vi "Stoerungen (129-192)- Messgeraet.vi"(8 "Fehler (Eingang)":errorcluster caption="Fehler (Eingang, kein Fehler)") -> (0 "Fehler (Ausgang)":errorcluster, 3 "Störungen 129-192":u64)   [LabVIEW 2020, in "Stoerungen.lvlib"]
uses:
  Stoerungen.lvlib
  Seiten/FT-IR/FGV FT-IR Diagnose Aktionen.ctl
  cRIO/Stoermeldungen/Stoerungen 129-192.ctl
  Aktionen Kommunikation Stoerung.ctl
  Seiten/Anlagengrenzwerte/Anlagen-Parameternamen.ctl
  Seiten/Erweiterte Konfig/FGV PID Aktionen.ctl
  Seiten/FT-IR/FGV FT-IR Aktionen.ctl
  Seiten/Log Konfig/Aktionen LogFile schreiben.ctl
  Funktionstasten/Funktionstasten-Aktion.ctl
  Funktionstasten/Zustaende.ctl
  Status Analysatoren/Aktion Status Analysatoren.ctl
  Seiten/EL3000/PMA/Aktion FGV Messwerte.ctl
  Seiten/EL3000/FID/Aktion FGV Messwerte_F.ctl
  Allgemein/Aktion FGV Aufheizphase.ctl
  Seiten/Lambdasonde/FGV Status Lambda Aktionen.ctl
  Seiten/FT-IR/FT-IR.lvlib
  cRIO/Stoermeldungen/Stoermeldungen.lvlib
  Seiten/Anlagengrenzwerte/Anlagengrenzwerte.lvlib
  Seiten/Erweiterte Konfig/Erweiterte Konfig.lvlib
  Seiten/Log Konfig/LogKonfig.lvlib
  cRIO/PC/Kommunikation mit cRIO.lvlib
  Funktionstasten/Funktionstasten.lvlib
  Status Analysatoren/Status Analysatoren.lvlib
  Seiten/EL3000/PMA/PMA.lvlib
  Seiten/EL3000/FID/FID.lvlib
  Seiten/Lambdasonde/Lambda_ Komm.lvlib
  Allgemein/allgemeine Sub-VIs.lvlib
panel:
  # "Störmeldungen Messgerät (129-192)"
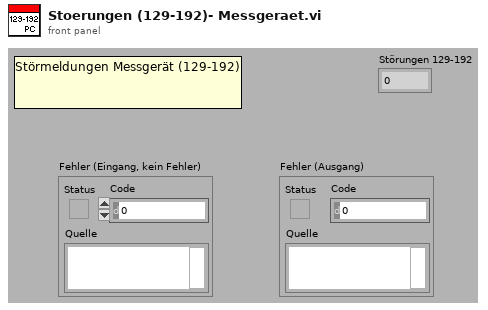
[diagram p1: front panel]
types:
  T1 = typedef "allgemeine Sub-VIs.lvlib/Aktion FGV Aufheizphase.ctl" = enum16{"init", "lesen", "PNS Filterblock", "PNS HL1", "PNS HL2", "PNS HL3", "PNS HL4", "FTIR Messzelle", "HL 1", "HL 2", "HL zu FTIR", "auswerten"}
  T2 = typedef "Status Analysatoren.lvlib/Aktion Status Analysatoren.ctl" = enum16{"lesen", "initialisieren", "Analysatoren aktiv", "FTIR Fehler", "FID Fehler", "PMA Fehler", "Felder einfärben"}
  T3 = typedef "ABB-EL3000.lvlib/FID.lvlib/Aktion FGV Messwerte_F.ctl" = enum16{"lesen", "Messwerte", "Messbereich", "Status", "Diagnose Werte"}
  T4 = typedef "ABB-EL3000.lvlib/PMA.lvlib/Aktion FGV Messwerte.ctl" = enum16{"lesen", "Messwerte", "Messbereich", "Status", "Diagnose Werte"}
  T5 = typedef "Funktionstasten.lvlib/Zustaende.ctl" = enum16{"Standby", "Pause", "Eco", "Messen", "Kalibrieren", "Spülen Filter", "Spülen Leitung", "Umgebungsluft", "0-Gas", "Cal-Gas", "CG zu PNS", "-------------", "Init 1", "Init 2", "Init 3", "Init 4", "Messen vorbereiten", "Messen durchführen", "Exit"}
  T6 = typedef "Funktionstasten.lvlib/Funktionstasten-Aktion.ctl" = enum16{"Initialisieren", "Zustand setzen", "Taste gedrückt", "Fehler speichern", "Lesen", "Manuell", "Remote", "Bitparallel", "Samplepoint", "Zeit Prüfen", "reset Umschalten"}
  T7 = typedef "LogKonfig.lvlib/Aktionen LogFile schreiben.ctl" = enum16{"lesen", "schreiben", "initialisieren"}
  T8 = typedef "FT-IR.lvlib/FGV FT-IR Aktionen.ctl" = enum16{"lesen", "NOG setzen", "NOS setzen", "Initialisieren", "speichern", "ALLES setzen", "FT-IR Spektrum loggen", "Komm Stoppen", "Spektrum LogKonfig"}
  T9 = typedef "Erweiterte Konfig.lvlib/FGV PID Aktionen.ctl" = enum16{"Lesen", "Schreiben PID", "Schreiben Sonstige", "Dichtheitstest", "Aktionen Dicht.", "Parameter Sensor"}
  T10 = typedef "Stoerungen.lvlib/Aktionen Kommunikation Stoerung.ctl" = enum16{"lesen", "init", "FT-IR Komm", "FT-IR Betriebsart", "FT-IR Hintergrund", "cRIO Komm", "PNS Komm", "Dichtheitstest", "Life Bit", "FTIR Komm AK", "PMA Komm", "FID Komm", "PMA Cal", "FID Ch4 Cal", "FID THC Cal", "Cal Timeout", "VFS 1 Komm", "VFS 2 Komm", "VFS 3 Komm", "VFS 4 Komm", "TRE 08 Komm", "CG-Test vorzeitig", "CG-Test Span 1", "CG-Test Span 2", "CG-Test Span 3", "CG-Test Messgas", "CG-Test löschen", "Test", "Amium AK", "AK Recept konfig", "AK Name konfig", "AK EKFG konfig"}
  T11 = typedef "Anlagengrenzwerte.lvlib/Anlagen-Parameternamen.ctl" = enum16{"Eingangsdruck FT-IR:", "Durchfluss FT-IR:", "Durchfluss CalGas", "Druck Ausgang", "Druck Kalter Block", "Heizleitung intern", "Heizleitung zu FT-IR", "Heizung Filter:", "Heizung Pumpe:", "HL Extern SP1", "HL Extern SP2", "FT-IR Messzelle", "Schaltschrank", "Gaskühler"}
  T12 = typedef "Stoermeldungen.lvlib/Stoerungen 129-192.ctl" = cluster{"ERR. 129":bool, "ERR. 130":bool, "ERR. 131":bool, "ERR. 132":bool, "ERR. 133":bool, "ERR. 134":bool, "ERR. 135":bool, "ERR. 136":bool, "ERR. 137":bool, "ERR. 138":bool, "ERR. 139":bool, "ERR. 140":bool, "ERR. 141":bool, "ERR. 142":bool, "ERR. 143":bool, "ERR. 144":bool, "ERR. 145":bool, "ERR. 146":bool, "ERR. 147":bool, "ERR. 148":bool, "ERR. 149":bool, "ERR. 150":bool, "ERR. 151":bool, "ERR. 152":bool, "ERR. 153":bool, "ERR. 154":bool, "ERR. 155":bool, "ERR. 156":bool, "ERR. 157":bool, "ERR. 158":bool, "ERR. 159":bool, "ERR. 160":bool, "ERR. 161":bool, "ERR. 162":bool, "ERR. 163":bool, "ERR. 164":bool, "ERR. 165":bool, "ERR. 166":bool, "ERR. 167":bool, "ERR. 168":bool, "ERR. 169":bool, "ERR. 170":bool, "ERR. 171":bool, "ERR. 172":bool, "ERR. 173":bool, "ERR. 174":bool, "ERR. 175":bool, "ERR. 176":bool, "ERR. 177":bool, "ERR. 178":bool, "ERR. 179":bool, "ERR. 180":bool, "ERR. 181":bool, "ERR. 182":bool, "ERR. 183":bool, "ERR. 184":bool, "ERR. 185":bool, "ERR. 186":bool, "ERR. 187":bool, "ERR. 188":bool, "ERR. 189":bool, "ERR. 190":bool, "ERR. 191":bool, "ERR. 192":bool}
  T13 = typedef "FT-IR.lvlib/FGV FT-IR Diagnose Aktionen.ctl" = enum16{"Lesen", "Diagnose Schreiben", "Min Schreiben", "Max Schreiben"}
  T14 = typedef "Stoerungen.lvlib/Stoerungen Messgeraete.ctl" = cluster{"FT-IR Komm":bool, "FT-IR Betriebsart":bool, "FT-IR Hintergrundscan":bool, "Dichtheitstest":bool, "cRIO Komm":bool, "PNS Komm":bool, "Life Bit":bool, "FT-IR AK Komm":bool, "PMA Komm":bool, "FID Komm":bool, "PMA Cal":bool, "FID CH4 Cal":bool, "FID THC Cal":bool, "Cal Timeout":bool, "VFS 1 Komm":bool, "VFS 2 Komm":bool, "VFS 3 Komm":bool, "VFS 4 Komm":bool, "TRE 08 Komm":bool, "CG-Test":bool, "CG-Test 1":bool, "CG-Test 2":bool, "CG-Test 3":bool, "Messgas - Eingang":bool, "Amium AK Komm":bool, "AK Rezept nicht konfiguriert ":bool, "AK Name nicht konfiguriert":bool, "AK EKFG nicht konfiguriert":bool}
  T15 = cluster{"LaserPP Max":dbl, "LinCheck Max":dbl, "sBeam Max":dbl}
  T16 = cluster{"LaserPP Min":dbl, "LinCheck Min":dbl, "sBeam Min":dbl}
  T17 = typedef "FT-IR.lvlib/TOOLweb Interface.lvlib/Typdefinitionen.lvlib/TOOLweb Diagnose.ctl" = cluster{"(14) temperature":sgl, "(15) pressure":sgl, "(16) oxygen":sgl, "(50) diag-igramdc":sgl, "(51) diag-igrampp":sgl, "(52) diag-phaseAngle":sgl, "(53) diag-laserpp":sgl, "(54) diag-laserdc":sgl, "(55) diag-badscan":sgl, "(56) diag-centerburst":sgl, "(57) diag-linearizerCheck":sgl, "(58) diag-SNR":sgl, "(59) diag-sBeamIntensity":sgl}
  T18 = typedef "Verwaltung - cRIO.lvlib/Digital Eingaenge 0-15.ctl" = cluster{"I0: N2 Nachf. FT-IR voll":bool, "I1: N2 Nachf. Vorrat leer":bool, "I2: (Klimaanlage eingeschaltet)":bool, "I3: (Klimaanlage Störung)":bool, "I4: Trigger Eingang (Messdaten sp.)":bool, "I5: Reserve":bool, "I6: Reserve":bool, "I7: Reserve":bool, "I8: Druckschalter Versorgung ok":bool, "I9: Reserve":bool, "I10: Reserve":bool, "I11: Reserve":bool, "I12: Drucksch. N2 Versorgung":bool, "I13: Reserve":bool, "I14: Drucksch. N2 Optikbox":bool, "I15: (Füllstand Kondensatbehälter)":bool}
  T19 = typedef "Status Analysatoren.lvlib/Status.ctl" = cluster{"FT-IR aktiv":bool, "FT-IR Fehler":bool, "FID aktiv":bool, "FID Fehler":bool, "PMA aktiv":bool, "PMA Fehler":bool}
  T20 = cluster{"Temperatur Detektor":sgl, "STG Detektor":sgl, "Temperatur MGE":sgl, "STG MGE":sgl, "Druck Brennluft":sgl, "STG Brennluft":sgl, "Druck Brenngas":sgl, "STG Brenngas":sgl, "Druck MGE":sgl, "STG Druck MGE":sgl, "Druck MGA":sgl, "STG Druck MGA":sgl, "Flow":sgl, "Temperatur Flamme":sgl, "Temperatur NMHC":sgl, "STG NMHC":sgl}
  T21 = cluster{"Ausfall":bool, "Funktionskontrolle":bool, "Wartungsbedarf":bool}
  T22 = cluster{"Temp. Detektor":sgl, "Temp. Regler":sgl, "STG Regler":sgl, "Druck Detektor":sgl}
  T23 = typedef "Erweiterte Konfig.lvlib/Sonstige Parameter.ctl" = cluster{"Lüfter langsam":sgl, "Lüfter schnell":sgl, "FT-IR Kühlung Soll":sgl, "FT-IR Kühlung Max":sgl, "Überwachung":T24, "Befüllung aktiv":T25, "Stickstoff Befüllzeit":sgl, "Befüllintervall":sgl, "Kalibrierwert FT-IR":sgl, "Offset Ausgang":sgl, "Offset FT-IR":sgl, "Offset Druck FT-IR":sgl, "Dichtheitstest Zeit":sgl, "Dichtheitstest Abfall":sgl, "Dichtheitstest Umfang":T26, "Offset Umgebung":sgl, "Max Taupunkt":sgl, "Pumpendrehzahl":sgl, "ext. Befüllung":T25, "Ext. Stickstoff Befüllzeit":sgl}
  T24 = typedef "Auswahlfeld.ctl" = u16
  T25 = typedef "LogKonfig.lvlib/Auswahlfeld aktiviert-deaktiviert.ctl" = u16
  T26 = typedef "Erweiterte Konfig.lvlib/Dichtheitstest Umfang.ctl" = u16
  T27 = typedef "Lambda_ Komm.lvlib/FGV Status Lambda Aktionen.ctl" = enum16{"lesen", "init", "Istwerte"}
  T28 = typedef "Lambda_ Komm.lvlib/Lambda Fehler.ctl" = cluster{"Komm":bool, "Lambda  Fehler":bool, "Ri Fehler":bool, "O2 Fehler":bool, "A/F Fehler":bool}
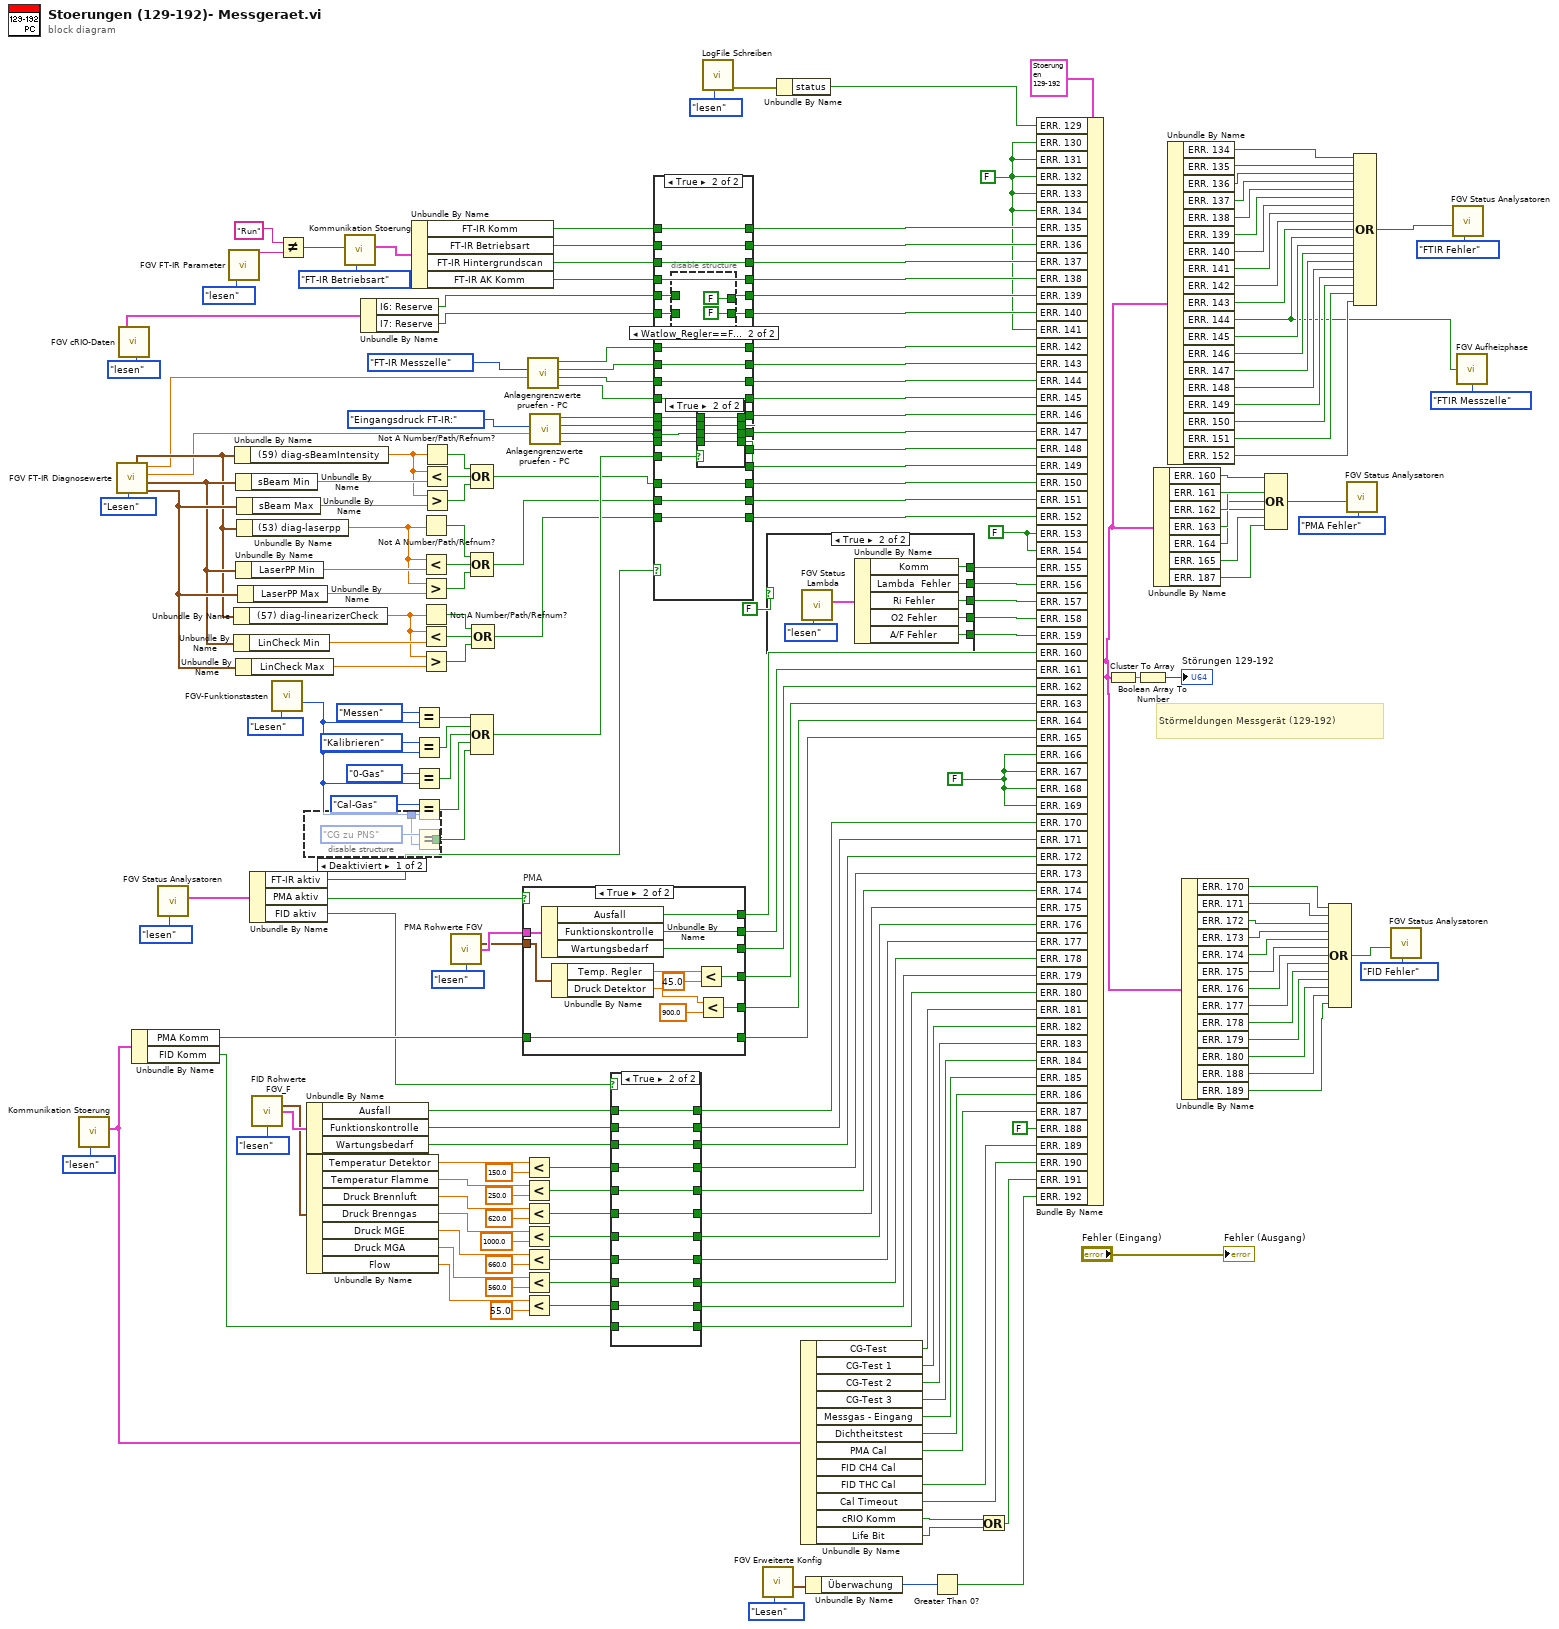
[diagram p0: block diagram]
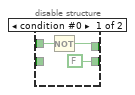
[diagram p7: hidden frame]
diagram:
  w16 = FALSE ("ERR. 173")
  w119 = FALSE ("ERR. 129")
  w67 = FALSE ("ERR. 129")
  # "Störmeldungen Messgerät (129-192)"
  n1 = call "Kommunikation Stoerung.vi"("Aktionen"=Aktionen_Kommunikation_Stoerung."lesen") -> ("Störung Messgerät"=w109:T14)  [unwired: 10 in]
  n2 = call "FGV FT-IR Diagnosewerte.vi"("Aktionen"=FGV_FT-IR_Diagnose_Aktionen."Lesen") -> ("FT-IR MAX"=w212:T15, "FT-IR MIN"=w211:T16, "Druck"=w202:dbl, "Temperatur"=w203:dbl, "Diagnose"=w210:T17)  [unwired: 5 in, 1 out]
  n3 = call "FGV cRIO-Daten.vi"("Aktion"=enum16{"lesen", "schreiben"}."lesen") -> ("DI"=w171:T18)  [unwired: 9 in, 9 out]
  n4 = Unbundle By Name(w109) -> ("PMA Komm"=w108:bool, "FID Komm"=w79:bool)
  n5 = call "FGV Status Analysatoren.vi"("Aktionen"=Aktion_Status_Analysatoren."lesen") -> ("Status Analysatoren"=w121:T19)  [unwired: 10 in]
  n6 = call "FGV FT-IR Parameter.vi"("Aktion"=FGV_FT-IR_Aktionen."lesen") -> ("Instrument State"=w189:string)  [unwired: 11 in, 7 out]
  n7 = Unbundle By Name(w210) -> ("(57) diag-linearizerCheck"=w178:sgl)
  n8 = Unbundle By Name(w211) -> ("LinCheck Min"=w206:dbl)
  n9 = Unbundle By Name(w210) -> ("(59) diag-sBeamIntensity"=w184:sgl)
  n10 = Unbundle By Name(w211) -> ("sBeam Min"=w214:dbl)
  n11 = Unbundle By Name(w211) -> ("LaserPP Min"=w209:dbl)
  n12 = Unbundle By Name(w212) -> ("LinCheck Max"=w207:dbl)
  n13 = Unbundle By Name(w212) -> ("sBeam Max"=w215:dbl)
  n14 = Unbundle By Name(w210) -> ("(53) diag-laserpp"=w179:sgl)
  n15 = Unbundle By Name(w212) -> ("LaserPP Max"=w208:dbl)
  n16 = Unbundle By Name(w121) -> ("FT-IR aktiv"=w120:bool, "PMA aktiv"=w21:bool, "FID aktiv"=w80:bool)
  n17 = call "FID Rohwerte FGV_F.vi"("Aktion"=Aktion_FGV_Messwerte_F."lesen") -> ("Diagnose Werte"=w102:T20, "Status"=w106:T21)  [unwired: 11 in, 2 out]
  n18 = call "FGV-Funktionstasten.vi"("Aktion"=Funktionstasten-Aktion."Lesen") -> ("ausgewählte Funktion"=w3:T5)  [unwired: 7 in, 7 out]
  n19 = Not Equal?(x="Run" ("y"), y=w189) -> (x != y?=w188:bool)
  n20 = disable-structure shown="Deaktiviert" {
    disable-tunnel: w3 -> [w218 _]
    disable-tunnel: [w217 _] -> w156
    frame Disabled {
      n21 = Equal?(x=Zustaende."CG zu PNS", y=w218) -> (x = y?=w217:bool)
    }
    frame Enabled {
    }
  }
  n22 = Unbundle By Name(w106) -> ("Ausfall"=w105:bool, "Funktionskontrolle"=w104:bool, "Wartungsbedarf"=w103:bool)
  n23 = Unbundle By Name(w102) -> ("Temperatur Detektor"=w101:sgl, "Temperatur Flamme"=w100:sgl, "Druck Brennluft"=w99:sgl, "Druck Brenngas"=w98:sgl, "Druck MGE"=w97:sgl, "Druck MGA"=w96:sgl, "Flow"=w95:sgl)
  n24 = call "Kommunikation Stoerung.vi"("Aktionen"=Aktionen_Kommunikation_Stoerung."FT-IR Betriebsart", "ERROR"=w188) -> ("Störung Messgerät"=w199:T14)  [unwired: 9 in]
  n25 = Unbundle By Name(w171) -> ("I6: Reserve"=w170:bool, "I7: Reserve"=w169:bool)
  n26 = Unbundle By Name(w199) -> ("FT-IR Komm"=w155:bool, "FT-IR Betriebsart"=w153:bool, "FT-IR Hintergrundscan"=w151:bool, "FT-IR AK Komm"=w149:bool)
  n27 = Equal?(x=Zustaende."Messen", y=w3) -> (x = y?=w160:bool)
  n28 = Equal?(x=Zustaende."Kalibrieren", y=w3) -> (x = y?=w159:bool)
  n29 = Equal?(x=Zustaende."0-Gas", y=w3) -> (x = y?=w158:bool)
  n30 = Equal?(x=Zustaende."Cal-Gas", y=w3) -> (x = y?=w157:bool)
  n31 = Not A Number/Path/Refnum?(number/path/refnum=w179) -> (NaN/Path/Refnum?=w183:bool)
  n32 = Less?(x=w179, y=w209) -> (x < y?=w182:bool)
  n33 = Greater?(x=w179, y=w208) -> (0:w176:bool)
  n34 = Not A Number/Path/Refnum?(number/path/refnum=w178) -> (NaN/Path/Refnum?=w181:bool)
  n35 = Less?(x=w178, y=w206) -> (x < y?=w180:bool)
  n36 = Greater?(x=w178, y=w207) -> (0:w177:bool)
  n37 = Not A Number/Path/Refnum?(number/path/refnum=w184) -> (NaN/Path/Refnum?=w185:bool)
  n38 = Less?(x=w184, y=w214) -> (x < y?=w187:bool)
  n39 = Greater?(x=w184, y=w215) -> (0:w186:bool)
  n40 = call "PMA Rohwerte FGV.vi"("Aktion"=Aktion_FGV_Messwerte."lesen") -> ("Diagnose Werte"=w116:T22, "Status"=w117:T21)  [unwired: 11 in, 2 out]
  n41 = Compound Arithmetic op=OR(w185, w187, w186) -> (w127:bool)
  n42 = Compound Arithmetic op=OR(w183, w182, w176) -> (w125:bool)
  n43 = Compound Arithmetic op=OR(w160, w159, w158, w157, w156) -> (w133:bool)
  n44 = Compound Arithmetic op=OR(w181, w180, w177) -> (w123:bool)
  n45 = case "PMA" shown="True" w21 {
    tunnel: w117 -> [_ w231]
    tunnel: w116 -> [_ w230]
    tunnel: [_ w225] -> w112
    tunnel: [_ w224] -> w111
    tunnel: [_ w223] -> w115
    tunnel: [_ w222] -> w114
    tunnel: [_ w221] -> w113
    tunnel: w108 -> [_ w220]
    tunnel: [_ w220] -> w110
    frame False {
    }
    frame True {
      n46 = Unbundle By Name(w231) -> ("Ausfall"=w223:bool, "Funktionskontrolle"=w222:bool, "Wartungsbedarf"=w221:bool)
      n47 = Unbundle By Name(w230) -> ("Temp. Regler"=w229:sgl, "Druck Detektor"=w226:sgl)
      n48 = Less?(x=w229, y=sgl 45.0) -> (x < y?=w225:bool)
      n49 = Less?(x=w226, y=sgl 900.0) -> (x < y?=w224:bool)
    }
  }
  n50 = Less?(x=w101, y=sgl 150.0) -> (x < y?=w87:bool)
  n51 = Less?(x=w100, y=sgl 250.0) -> (x < y?=w86:bool)
  n52 = Less?(x=w99, y=sgl 620.0) -> (x < y?=w85:bool)
  n53 = Less?(x=w98, y=sgl 1000.0) -> (x < y?=w84:bool)
  n54 = Less?(x=w97, y=sgl 660.0) -> (x < y?=w83:bool)
  n55 = Less?(x=w96, y=sgl 560.0) -> (x < y?=w82:bool)
  n56 = Less?(x=w95, y=sgl 55.0) -> (x < y?=w81:bool)
  n57 = call "Anlagengrenzwerte pruefen - PC.vi"("Wert"=w203, "Anlagen-Parametername"=Anlagen-Parameternamen."FT-IR Messzelle") -> ("AbschMax"=w138:bool, "AbschMin"=w140:bool, "WarnMax"=w142:bool, "WarnMin"=w144:bool)  [unwired: 5 in, 1 out]
  n58 = call "Anlagengrenzwerte pruefen - PC.vi"("Wert"=w202, "Anlagen-Parametername"=Anlagen-Parameternamen."Eingangsdruck FT-IR:") -> ("AbschMax"=w134:bool, "AbschMin"=w135:bool, "WarnMax"=w137:bool, "WarnMin"=w136:bool)  [unwired: 5 in, 1 out]
  n59 = case shown="True" w80 {
    tunnel: w105 -> [_ w237]
    tunnel: w104 -> [_ w236]
    tunnel: w103 -> [_ w235]
    tunnel: w87 -> [_ w234]
    tunnel: w86 -> [_ w233]
    tunnel: w85 -> [_ w232]
    tunnel: w84 -> [_ w238]
    tunnel: w83 -> [_ w239]
    tunnel: w82 -> [_ w240]
    tunnel: w81 -> [_ w241]
    tunnel: w79 -> [_ w242]
    tunnel: [_ w242] -> w68
    tunnel: [_ w241] -> w69
    tunnel: [_ w240] -> w70
    tunnel: [_ w239] -> w71
    tunnel: [_ w238] -> w72
    tunnel: [_ w237] -> w78
    tunnel: [_ w236] -> w77
    tunnel: [_ w235] -> w76
    tunnel: [_ w234] -> w75
    tunnel: [_ w233] -> w74
    tunnel: [_ w232] -> w73
    frame False {
    }
    frame True {
    }
  }
  n60 = case shown="True" w120 {
    tunnel: w155 -> [_ w266]
    tunnel: [_ w266] -> w154
    tunnel: w153 -> [_ w265]
    tunnel: [_ w265] -> w152
    tunnel: w151 -> [_ w264]
    tunnel: [_ w264] -> w150
    tunnel: w149 -> [_ w263]
    tunnel: [_ w263] -> w148
    tunnel: w170 -> [_ w244]
    tunnel: [_ w246] -> w147
    tunnel: w169 -> [_ w243]
    tunnel: [_ w245] -> w146
    tunnel: [_ w262] -> w145
    tunnel: w144 -> [_ w262]
    tunnel: w142 -> [_ w261]
    tunnel: [_ w261] -> w143
    tunnel: [_ w260] -> w141
    tunnel: w140 -> [_ w260]
    tunnel: [_ w259] -> w139
    tunnel: w138 -> [_ w259]
    tunnel: w136 -> [_ w258]
    tunnel: w137 -> [_ w257]
    tunnel: w135 -> [_ w256]
    tunnel: w134 -> [_ w255]
    tunnel: w133 -> [_ w254]
    tunnel: [_ w253] -> w132
    tunnel: [_ w252] -> w131
    tunnel: [_ w251] -> w130
    tunnel: [_ w250] -> w129
    tunnel: [_ w249] -> w128
    tunnel: w127 -> [_ w249]
    tunnel: [_ w248] -> w126
    tunnel: w125 -> [_ w248]
    tunnel: [_ w247] -> w124
    tunnel: w123 -> [_ w247]
    frame False {
    }
    frame True {
      n61 = disable-structure shown="Watlow_Regler==FALSE, Standard" {
        disable-tunnel: [w268 FALSE] -> w246
        disable-tunnel: [FALSE FALSE] -> w245
        disable-tunnel: w244 -> [w269 _]
        disable-tunnel: w243 -> [_ _]
        frame condition #0 {
          n62 = Not(x=w269) -> (.not. x?=w268:bool)
        }
        frame condition #1 (active) {
        }
      }
      n63 = case shown="True" w254 {
        tunnel: w258 -> [_ w272]
        tunnel: w257 -> [_ w273]
        tunnel: w256 -> [_ w274]
        tunnel: w255 -> [_ w275]
        tunnel: [_ w275] -> w250
        tunnel: [_ w274] -> w251
        tunnel: [_ w273] -> w252
        tunnel: [_ w272] -> w253
        frame False {
        }
        frame True {
        }
      }
    }
  }
  n64 = call "LogFile Schreiben.vi"("Aktion"=Aktionen_LogFile_schreiben."lesen") -> ("error out"=w173:errorcluster)  [unwired: 7 in, 3 out]
  n65 = call "FGV Erweiterte Konfig.vi"("Aktion"=FGV_PID_Aktionen."Lesen") -> ("Sonstige"=w195:T23)  [unwired: 6 in, 4 out]
  n66 = case shown="True" FALSE {
    tunnel: [_ w280] -> w66
    tunnel: [_ w279] -> w65
    tunnel: [_ w278] -> w64
    tunnel: [_ w277] -> w63
    tunnel: [_ w276] -> w62
    frame False {
    }
    frame True {
      n67 = call "FGV Status Lambda.vi"("Aktionen"=FGV_Status_Lambda_Aktionen."lesen") -> ("Lambda Fehler"=w282:T28)  [unwired: 9 in, 1 out]
      n68 = Unbundle By Name(w282) -> ("Komm"=w280:bool, "Lambda  Fehler"=w279:bool, "Ri Fehler"=w278:bool, "O2 Fehler"=w277:bool, "A/F Fehler"=w276:bool)
    }
  }
  n69 = Unbundle By Name(w173) -> ("status"=w175:bool)
  n70 = Unbundle By Name(w109) -> ("CG-Test"=w11:bool, "CG-Test 1"=w12:bool, "CG-Test 2"=w13:bool, "CG-Test 3"=w14:bool, "Messgas - Eingang"=w15:bool, "Dichtheitstest"=w17:bool, "PMA Cal"=w10:bool, "FID THC Cal"=w18:bool, "Cal Timeout"=w19:bool, "cRIO Komm"=w168:bool, "Life Bit"=w167:bool)  [unwired: 1 out]
  n71 = Unbundle By Name(w195) -> ("Überwachung"=w193:T24)
  n72 = Greater Than 0?(x=w193) -> (x > 0?=w192:bool)
  n73 = Or(x=w168, y=w167) -> (x .or. y?=w166:bool)
  n74 = Bundle By Name(cluster=T12 {"ERR. 129"=FALSE, "ERR. 130"=FALSE, "ERR. 131"=FALSE, "ERR. 132"=FALSE, "ERR. 133"=FALSE, "ERR. 134"=FALSE, "ERR. 135"=FALSE, "ERR. 136"=FALSE, "ERR. 137"=FALSE, "ERR. 138"=FALSE, "ERR. 139"=FALSE, "ERR. 140"=FALSE, "ERR. 141"=FALSE, "ERR. 142"=FALSE, "ERR. 143"=FALSE, "ERR. 144"=FALSE, "ERR. 145"=FALSE, "ERR. 146"=FALSE, "ERR. 147"=FALSE, "ERR. 148"=FALSE, "ERR. 149"=FALSE, "ERR. 150"=FALSE, "ERR. 151"=FALSE, "ERR. 152"=FALSE, "ERR. 153"=FALSE, "ERR. 154"=FALSE, "ERR. 155"=FALSE, "ERR. 156"=FALSE, "ERR. 157"=FALSE, "ERR. 158"=FALSE, "ERR. 159"=FALSE, "ERR. 160"=FALSE, "ERR. 161"=FALSE, "ERR. 162"=FALSE, "ERR. 163"=FALSE, "ERR. 164"=FALSE, "ERR. 165"=FALSE, "ERR. 166"=FALSE, "ERR. 167"=FALSE, "ERR. 168"=FALSE, "ERR. 169"=FALSE, "ERR. 170"=FALSE, "ERR. 171"=FALSE, "ERR. 172"=FALSE, "ERR. 173"=FALSE, "ERR. 174"=FALSE, "ERR. 175"=FALSE, "ERR. 176"=FALSE, "ERR. 177"=FALSE, "ERR. 178"=FALSE, "ERR. 179"=FALSE, "ERR. 180"=FALSE, "ERR. 181"=FALSE, "ERR. 182"=FALSE, "ERR. 183"=FALSE, "ERR. 184"=FALSE, "ERR. 185"=FALSE, "ERR. 186"=FALSE, "ERR. 187"=FALSE, "ERR. 188"=FALSE, "ERR. 189"=FALSE, "ERR. 190"=FALSE, "ERR. 191"=FALSE, "ERR. 192"=FALSE} ("STÖRUNGEN 129-192"), "ERR. 129"=w175, "ERR. 130"=w67, "ERR. 131"=w67, "ERR. 132"=w67, "ERR. 133"=w67, "ERR. 134"=w67, "ERR. 135"=w154, "ERR. 136"=w152, "ERR. 137"=w150, "ERR. 138"=w148, "ERR. 139"=w147, "ERR. 140"=w146, "ERR. 141"=w67, "ERR. 142"=w145, "ERR. 143"=w143, "ERR. 144"=w141, "ERR. 145"=w139, "ERR. 146"=w132, "ERR. 147"=w131, "ERR. 148"=w130, "ERR. 149"=w129, "ERR. 150"=w128, "ERR. 151"=w126, "ERR. 152"=w124, "ERR. 153"=w119, "ERR. 154"=w119, "ERR. 155"=w66, "ERR. 156"=w65, "ERR. 157"=w64, "ERR. 158"=w63, "ERR. 159"=w62, "ERR. 160"=w115, "ERR. 161"=w114, "ERR. 162"=w113, "ERR. 163"=w112, "ERR. 164"=w111, "ERR. 165"=w110, "ERR. 166"=w16, "ERR. 167"=w16, "ERR. 168"=w16, "ERR. 169"=w16, "ERR. 170"=w78, "ERR. 171"=w77, "ERR. 172"=w76, "ERR. 173"=w75, "ERR. 174"=w74, "ERR. 175"=w73, "ERR. 176"=w72, "ERR. 177"=w71, "ERR. 178"=w70, "ERR. 179"=w69, "ERR. 180"=w68, "ERR. 181"=w11, "ERR. 182"=w12, "ERR. 183"=w13, "ERR. 184"=w14, "ERR. 185"=w15, "ERR. 186"=w17, "ERR. 187"=w10, "ERR. 188"=FALSE, "ERR. 189"=w18, "ERR. 190"=w19, "ERR. 191"=w166, "ERR. 192"=w192) -> (w34:T12)
  n75 = Cluster To Array(cluster=w34) -> (array=w205:bool[])
  n76 = Boolean Array To Number ("Boolesches Array nach Zahl")(Boolean array=w205) -> (number=→"Störungen 129-192":u64)
  n77 = Unbundle By Name(w34) -> ("ERR. 160"=w60:bool, "ERR. 161"=w59:bool, "ERR. 162"=w58:bool, "ERR. 163"=w57:bool, "ERR. 164"=w56:bool, "ERR. 165"=w8:bool, "ERR. 187"=w7:bool)
  n78 = Unbundle By Name(w34) -> ("ERR. 134"=w53:bool, "ERR. 135"=w52:bool, "ERR. 136"=w51:bool, "ERR. 137"=w50:bool, "ERR. 138"=w49:bool, "ERR. 139"=w48:bool, "ERR. 140"=w47:bool, "ERR. 141"=w46:bool, "ERR. 142"=w45:bool, "ERR. 143"=w44:bool, "ERR. 144"=w1:bool, "ERR. 145"=w43:bool, "ERR. 146"=w42:bool, "ERR. 147"=w41:bool, "ERR. 148"=w40:bool, "ERR. 149"=w39:bool, "ERR. 150"=w38:bool, "ERR. 151"=w37:bool, "ERR. 152"=w6:bool)
  n79 = Unbundle By Name(w34) -> ("ERR. 170"=w33:bool, "ERR. 171"=w32:bool, "ERR. 172"=w31:bool, "ERR. 173"=w30:bool, "ERR. 174"=w29:bool, "ERR. 175"=w28:bool, "ERR. 176"=w27:bool, "ERR. 177"=w26:bool, "ERR. 178"=w25:bool, "ERR. 179"=w24:bool, "ERR. 180"=w23:bool, "ERR. 188"=w5:bool, "ERR. 189"=w4:bool)
  n80 = Compound Arithmetic op=OR ("Mehrfacharithmetik")(w60, w59, w58, w57, w56, w8, w7) -> (w55:bool)
  n81 = Compound Arithmetic op=OR ("Mehrfacharithmetik")(w33, w32, w31, w30, w29, w28, w27, w26, w25, w24, w23, w5, w4) -> (w22:bool)
  n82 = call "FGV Status Analysatoren.vi"("Aktionen"=Aktion_Status_Analysatoren."PMA Fehler", "Fehler"=w55) -> ()  [unwired: 9 in, 1 out]
  n83 = Compound Arithmetic op=OR ("Mehrfacharithmetik")(w53, w52, w51, w50, w49, w48, w47, w46, w45, w44, w1, w43, w42, w41, w40, w39, w38, w37, w6) -> (w36:bool)
  n84 = call "FGV Status Analysatoren.vi"("Aktionen"=Aktion_Status_Analysatoren."FID Fehler", "Fehler"=w22) -> ()  [unwired: 9 in, 1 out]
  n85 = call "FGV Status Analysatoren.vi"("Aktionen"=Aktion_Status_Analysatoren."FTIR Fehler", "Fehler"=w36) -> ()  [unwired: 9 in, 1 out]
  n86 = call "FGV Aufheizphase.vi"("Error"=w1, "Aktion"=Aktion_FGV_Aufheizphase."FTIR Messzelle") -> ()  [unwired: 11 in, 3 out]
  "Fehler (Ausgang)" <- "Fehler (Eingang)"
